vi "test.vi"   [LabVIEW 2010]
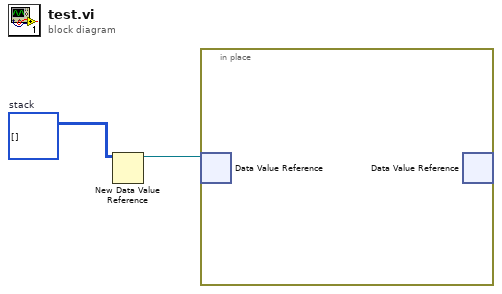
[diagram p0: block diagram]
diagram:
  w2 = i32[][][] []  # stack
  n1 = New Data Value Reference(data value=w2) -> (data value reference=w1:refnum<data-value>)  [unwired: 1 in, 1 out]
  n2 = in-place {
    n3 = in-place-dvr #1(w1) -> ()  [unwired: 2 out]
    n4 = in-place-dvr #1() -> ()  [unwired: 1 in, 2 out]
  }
